vi "Create From Variant.vi"(8 "error in (no error)":errorcluster, 10 "Variant":variant, 11 "JSON Object in":refnum<class "JSON Object.lvclass">) -> (0 "error out":errorcluster, 3 "JSON Object out":refnum<class "JSON Object.lvclass">)   [LabVIEW 2015, in "LVJSON.lvlib" / "JSON Object.lvclass"]
uses:
  JSON Object.lvclass
  JSON Numeric/JSON Numeric.lvclass
  JSON String/JSON String.lvclass
  JSON Boolean/JSON Boolean.lvclass
  JSON Array/JSON Array.lvclass
  JSON Null/JSON Null.lvclass
  Insert Key Value Pair (Multi).vi
  JSON String/New JSON String.vi
  <vilib>/Utility/Data Type/NI_Data Type.lvlib
  JSON Datatype/JSON Datatype.lvclass
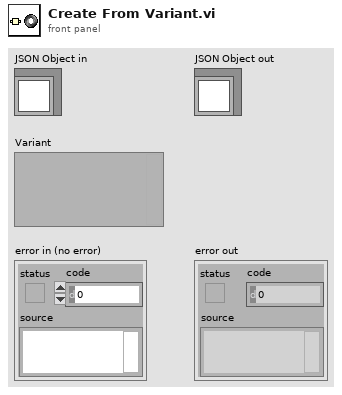
[diagram p1: front panel]
types:
  T1 = typedef "NI_Data Type.lvlib/Data Type.ctl" = enum8{"Invalid Type", "Void", "I8", "I16", "I32", "I64", "U8", "U16", "U32", "U64", "Single Float", "Double Float", "Extended Float", "Single Complex", "Double Complex", "Extended Complex", "Enum U8", "Enum U16", "Enum U32", "Enum U64", "Single Float With Unit", "Double Float With Unit", "Extended Float With Unit", "Single Complex with Unit", "Double Complex with Unit", "Extended Complex with Unit", "Boolean", "String", "Path", "Picture", "Tag", "Array", "Cluster", "Variant", "LV Variant", "Waveform", "Timestamp", "Digital Waveform", "Digital Data", "ExpressData", "Refnum", "External Data", "VI", "Poly VI", "LabVIEW Class Instance", "Fixed Point"}
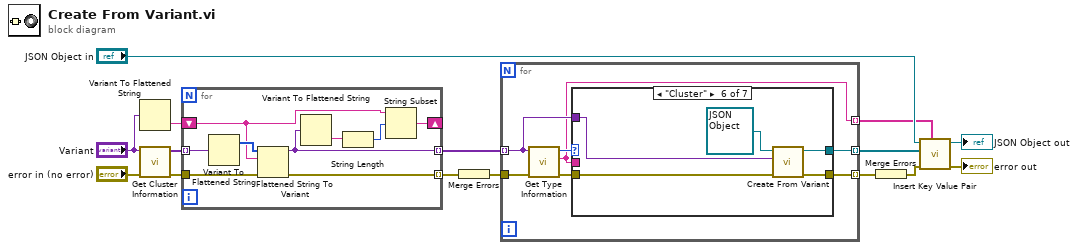
[diagram p0: block diagram]
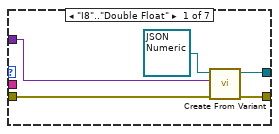
[diagram p2: hidden frame]
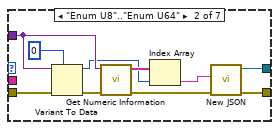
[diagram p3: hidden frame]
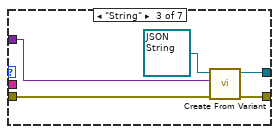
[diagram p4: hidden frame]
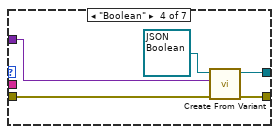
[diagram p5: hidden frame]
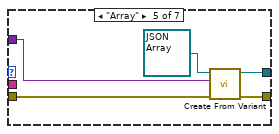
[diagram p6: hidden frame]
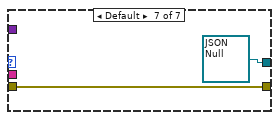
[diagram p7: hidden frame]
diagram:
  n1 = Variant To Flattened String(Variant="Variant") -> (data string=w15:string)  [unwired: 1 out]
  n2 = call <vilib>:"Get Cluster Information.vi"("error in (no error)"="error in (no error)", "Variant"="Variant") -> ("error out"=w12:errorcluster, "Cluster Elements"=w14:variant[])  [unwired: 8 in]
  n3 = for {
    tunnel: w14 -> [w24] mode=indexing
    tunnel: [w22] -> w13 mode=indexing
    shift-right: [w18] -> _
    shift-left: w15 -> [w21]
    tunnel: w12 -> [w17]
    tunnel: [w16] -> w11 mode=indexing
    n4 = Variant To Flattened String(Variant=w24) -> (1:w23:i16[])  [unwired: 1 out]
    n5 = Flattened String To Variant(4:w17, 6:w21, 7:w23) -> (0:w16:errorcluster, 3:w22:variant)
    n6 = Variant To Flattened String(Variant=w22) -> (data string=w20:string)  [unwired: 1 out]
    n7 = String Length(string=w20) -> (length=w19:i32)
    n8 = String Subset(string=w21, offset (0)=w19) -> (substring=w18:string)  [unwired: 1 in]
  }
  n9 = Merge Errors(w11) -> (w10:errorcluster)
  n10 = for {
    tunnel: w13 -> [w30] mode=indexing
    tunnel: [w29] -> w1 mode=indexing
    tunnel: [w28] -> w2 mode=indexing
    tunnel: w10 -> [w27]
    tunnel: [w25] -> w9 mode=indexing
    n11 = call <vilib>:"Get Type Information.vi"("error in (no error)"=w27, "Variant"=w30) -> ("error out"=w26:errorcluster, "Name"=w28:string, "Type"=w31:T1)  [unwired: 5 in, 2 out]
    n12 = case shown="\"Cluster\"" w31 {
      tunnel: w30 -> [w35 w44 w50 w55 w60 w65 _]
      tunnel: [w32 w46 w47 w52 w59 w62 refnum<class "JSON Null.lvclass"> refnum ("JSON String out")] -> w29
      tunnel: w28 -> [_ _ _ _ _ _ _]
      tunnel: w26 -> [w34 w39 w49 w54 w58 w64 w67]
      tunnel: [w33 w45 w48 w53 w57 w63 w67] -> w25
      frame "I8".."Double Float" {
        n13 = call-dynamic "Create From Variant.vi"("error in (no error)"=w34, "Variant"=w35, "JSON Numeric in"=refnum<class "JSON Numeric.lvclass"> refnum ("JSON Object in")) -> ("error out"=w33:errorcluster, "JSON Numeric out"=w32:refnum<class "JSON Numeric.lvclass">)  [unwired: 7 in]
      }
      frame "Enum U8".."Enum U64" {
        n14 = Variant To Data(error in=w39, type=u64 0, Variant=w44) -> (data=w41:u64, error out=w38:errorcluster)
        n15 = call <vilib>:"Get Numeric Information.vi"("error in (no error)"=w38, "Variant"=w44) -> ("error out"=w37:errorcluster, "Enum Names"=w42:string[])  [unwired: 6 in, 2 out]
        n16 = Index Array(array=w42, index=w41) -> (element=w40:string)
        n17 = call-poly "New JSON.vi"("error in (no error)"=w37, "value"=w40) -> ("error out"=w45:errorcluster, "JSON String out"=w46:refnum<class "JSON String.lvclass">)  [unwired: 8 in]
      }
      frame "String" {
        n18 = call-dynamic "Create From Variant.vi"("error in (no error)"=w49, "Variant"=w50, "JSON String in"=refnum<class "JSON String.lvclass"> refnum ("JSON Object in")) -> ("error out"=w48:errorcluster, "JSON String out"=w47:refnum<class "JSON String.lvclass">)  [unwired: 7 in]
      }
      frame "Boolean" {
        n19 = call-dynamic "Create From Variant.vi"("error in (no error)"=w54, "Variant"=w55, "JSON Boolean in"=refnum<class "JSON Boolean.lvclass"> refnum ("JSON Object in")) -> ("error out"=w53:errorcluster, "JSON Boolean out"=w52:refnum<class "JSON Boolean.lvclass">)  [unwired: 7 in]
      }
      frame "Array" {
        n20 = call-dynamic "Create From Variant.vi"("error in (no error)"=w58, "Variant"=w60, "JSON Array in"=refnum<class "JSON Array.lvclass"> refnum ("JSON Object in")) -> ("error out"=w57:errorcluster, "JSON Array out"=w59:refnum<class "JSON Array.lvclass">)  [unwired: 7 in]
      }
      frame "Cluster" {
        n21 = call-dynamic "Create From Variant.vi"("error in (no error)"=w64, "Variant"=w65, "JSON Object in"=refnum<class "JSON Object.lvclass"> refnum) -> ("error out"=w63:errorcluster, "JSON Object out"=w62:refnum<class "JSON Object.lvclass">)  [unwired: 7 in]
      }
      frame Default {
      }
    }
  }
  n22 = Merge Errors(w9) -> (w8:errorcluster)
  n23 = call-poly "Insert Key Value Pair.vi"("keys"=w2, "error in (no error)"=w8, "values"=w1, "JSON Object in"="JSON Object in") -> ("error out"=→"error out":errorcluster, "JSON Object out"=→"JSON Object out":refnum<class "JSON Object.lvclass">)  [unwired: 5 in, 1 out]
